vi "host_save_data.vi"(8 "error in":errorcluster) -> (0 "error out":errorcluster)   [LabVIEW 2021]
doc: "Save stored data."
uses:
  core/host_global_vars.vi
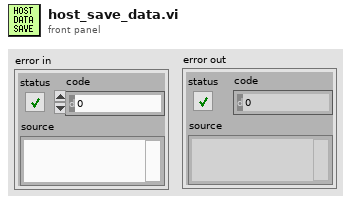
[diagram p1: front panel]
types:
  T1 = enum16{"open", "replace", "create", "open or create", "replace or create", "replace or create with confirmation"}
  T2 = enum16{"big-endian, network order", "native, host order", "little-endian"}
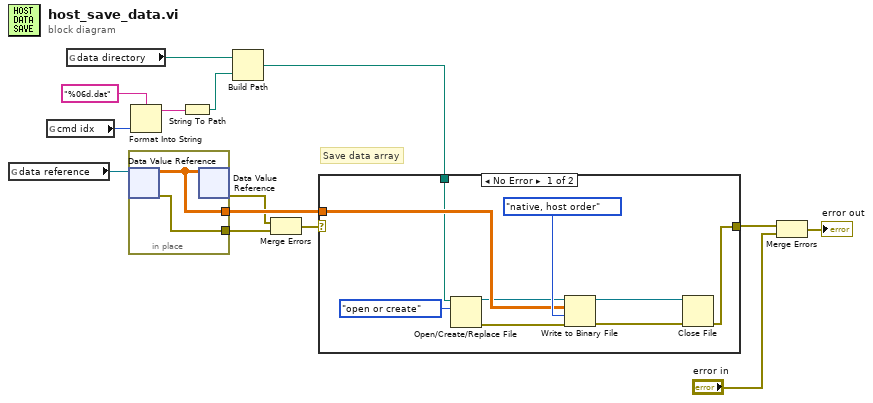
[diagram p0: block diagram]
diagram:
  # "Save data array"
  n1 = global read "host_global_vars.vi" "data reference"() -> (w14:refnum<data-value>)
  n2 = global read "host_global_vars.vi" "cmd idx"() -> (w5:i32)
  n3 = global read "host_global_vars.vi" "data directory"() -> (w6:path)
  n4 = in-place {
    in-place-border: [w16] -> w13
    in-place-border: [w15] -> w10
    n5 = in-place-dvr #1(w14) -> (w16:sgl[][][][], w15:errorcluster)
    n6 = in-place-dvr #1(w16) -> (w11:errorcluster)  [unwired: 1 out]
  }
  n7 = Format Into String(format string="%06d.dat", w5) -> (resulting string=w3:string)  [unwired: 2 in, 1 out]
  n8 = String To Path(string=w3) -> (path=w2:path)
  n9 = Build Path(base path=w6, name or relative path=w2) -> (appended path=w1:path)
  n10 = Merge Errors(w11, w10) -> (w12:errorcluster)
  n11 = case shown="No Error" w12 {
    selector: w12 -> [_ w26]
    tunnel: w13 -> [w24 _]
    tunnel: [w18 w26] -> w9
    tunnel: w1 -> [w17 _]
    frame No Error {
      n12 = Open/Create/Replace File(file path (use dialog)=w17, operation (0:open)=T1."open or create") -> (refnum out=w22:refnum<file>, error out=w23:errorcluster)  [unwired: 4 in, 1 out]
      n13 = Write to Binary File(file (use dialog)=w22, data=w24, error in=w23, 9:T2."native, host order" ("byte order (0:big-endian, network order)")) -> (refnum out=w20:refnum<file>, error out=w19:errorcluster)  [unwired: 2 in, 1 out]
      n14 = Close File(refnum=w20, error in=w19) -> (error out=w18:errorcluster)  [unwired: 1 out]
    }
    frame Error {
    }
  }
  n15 = Merge Errors(w9, "error in") -> (→"error out":errorcluster)
